vi "Read.vi"(8 "error in (no error)":errorcluster, 10 "ILC In":refnum<class "ILC.lvclass">, 11 "ILC ADC in":refnum<class "ILC ADC.lvclass">) -> (0 "error out":errorcluster, 1 "Value":dbl[unit], 2 "ILC Out":refnum<class "ILC.lvclass">, 3 "ILC ADC out":refnum<class "ILC ADC.lvclass">)   [LabVIEW 2015, in "ILC ADC.lvclass"]
uses:
  ILC ADC.lvclass
  <userlib>/Common/ILC/ILC/ILC.lvclass
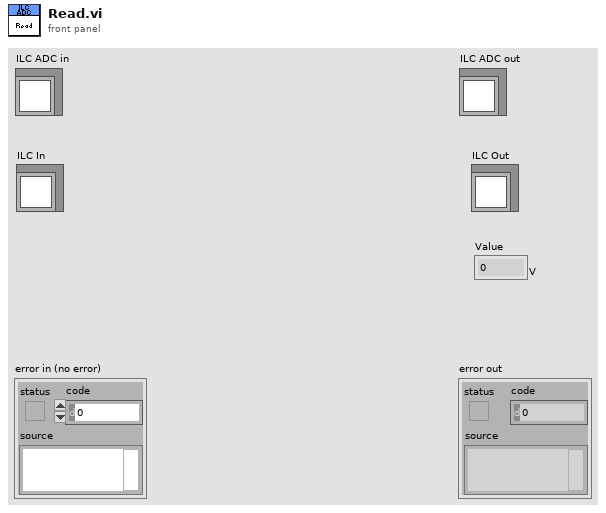
[diagram p1: front panel]
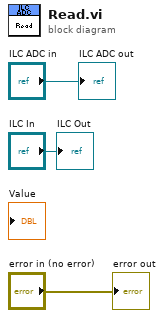
[diagram p0: block diagram]
diagram:
  "error out" <- "error in (no error)"
  "ILC ADC out" <- "ILC ADC in"
  "ILC Out" <- "ILC In"
